vi "GlobalSetNumberOfDigits_Scanners.vi"() -> ()   [LabVIEW 2011]
panel:
  in  "NumberOfDigits Scanner":i32=15 min=1 max=15 step=1
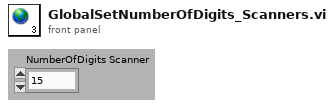
[diagram p1: front panel]
diagram:
